vi "12 Simulated DAQmx Signal.vi"() -> ()   [LabVIEW 2017]
uses:
  <vilib>/DAQmx/configure/timing.llb/DAQmx Timing (Sample Clock).vi
  <vilib>/DAQmx/configure/trigger.llb/DAQmx Trigger.vi
  <vilib>/DAQmx/configure/trigger.llb/DAQmx Start Trigger (Digital Edge).vi
panel:
  out "Waveform Chart":dynamicdata(graph)
  in  "stop (F)":bool
  out "error out":errorcluster
  out "task out":refnum<k21>
  in  "number of samples":i32=240
  in  "rate":dbl=6000.0
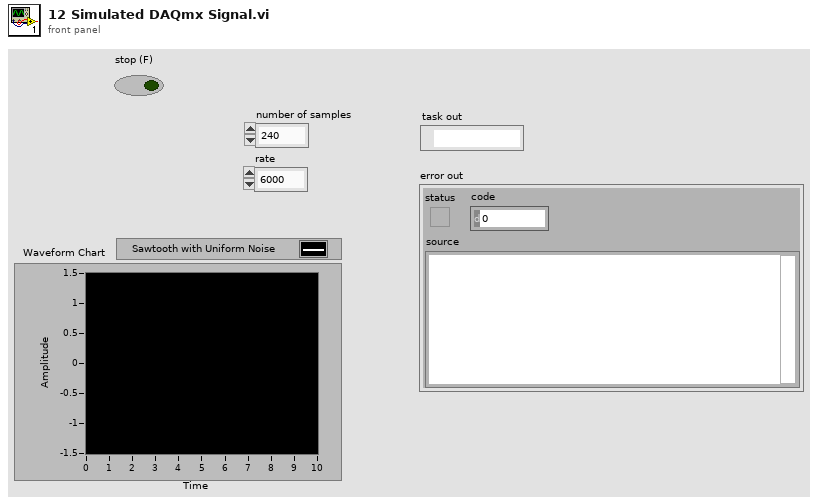
[diagram p1: front panel]
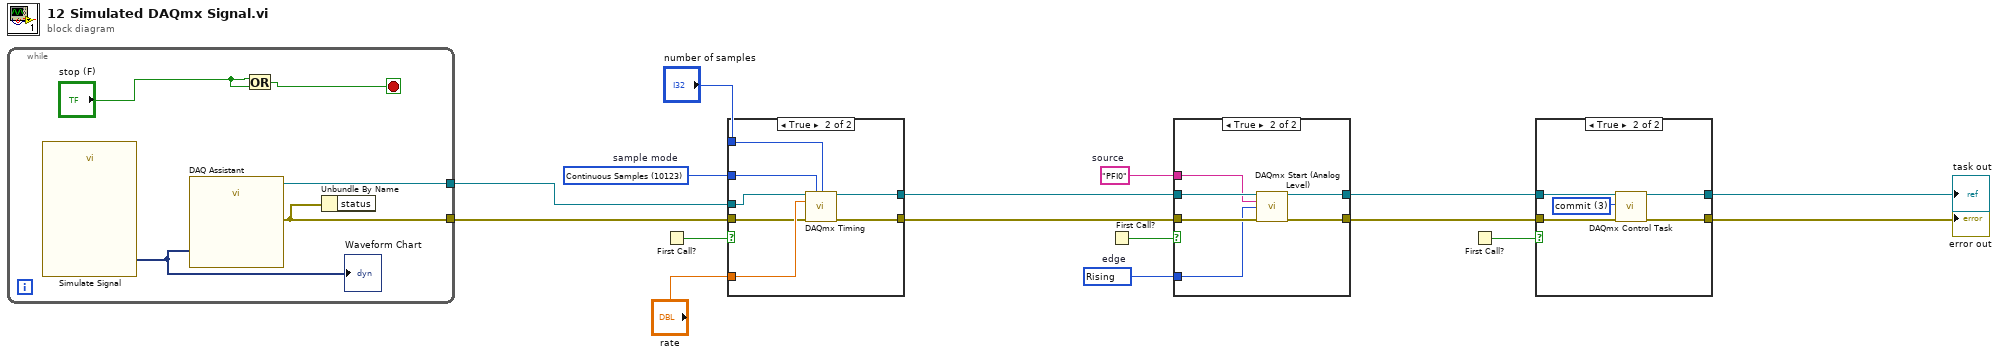
[diagram p0: block diagram]
diagram:
  w12 = 10280 items=["Rising"=10280, "Falling"=10171]  # edge
  w11 = "PFI0"  # source
  w7 = 10123 items=["Finite Samples"=10178, "Continuous Samples"=10123, "Hardware Timed Single Point"=12522]  # sample mode
  n1 = while {
    tunnel: [w20] -> w2
    tunnel: [w19] -> w1
    stop <- w21 stop-if-true
    n2 = call "Simulate Signal"() -> ("Sawtooth with Uniform Noise"=w18:dynamicdata)  [unwired: 14 in, 1 out]
    "Waveform Chart" <- w18
    n3 = call "DAQ Assistant"("data"=w18) -> ("task out"=w20:refnum<k21>, "error out"=w19:errorcluster)  [unwired: 16 in, 1 out]
    n4 = Or(x="stop (F)", y="stop (F)") -> (x .or. y?=w21:bool)
    n5 = Unbundle By Name(w19) -> ()  [unwired: 1 out]
  }
  n6 = First Call?() -> (First Call?: T/F=w3:bool)
  n7 = case shown="True" w3 {
    tunnel: [w23 w27] -> w9
    tunnel: [w22 w26] -> w4
    tunnel: "number of samples" -> [_ w30]
    tunnel: w7 -> [_ w29]
    tunnel: "rate" -> [_ w28]
    tunnel: w2 -> [w23 w25]
    tunnel: w1 -> [w22 w24]
    frame False {
    }
    frame True {
      n8 = call-poly <vilib>:"DAQmx Timing.vi"("task/channels in"=w25, "sample mode"=w29, "samples per channel"=w30, "rate"=w28, "error in"=w24) -> ("task out"=w27:refnum<k21>, "error out"=w26:errorcluster)  [unwired: 9 in]
    }
  }
  n9 = First Call?() -> (First Call?: T/F=w8:bool)
  n10 = case shown="True" w8 {
    tunnel: [w32 w36] -> w14
    tunnel: w9 -> [w32 w38]
    tunnel: [w31 w35] -> w10
    tunnel: w4 -> [w31 w37]
    tunnel: w11 -> [_ w34]
    tunnel: w12 -> [_ w33]
    frame False {
    }
    frame True {
      n11 = call-poly "DAQmx Start (Analog Level).vi"("task/channels in"=w38, "source"=w34, "edge"=w33, "error in"=w37) -> ("task out"=w36:refnum<k21>, "error out"=w35:errorcluster)  [unwired: 10 in]
    }
  }
  n12 = First Call?() -> (First Call?: T/F=w13:bool)
  n13 = case shown="True" w13 {
    tunnel: [w40 w44] -> w16
    tunnel: w14 -> [w40 w45]
    tunnel: [w39 w42] -> w15
    tunnel: w10 -> [w39 w43]
    frame False {
    }
    frame True {
      w41 = 3 items=["verify"=2, "reserve"=4, "commit"=3, "unreserve"=5, "abort"=6] ("action")
      n14 = call <vilib>:"DAQmx Control Task.vi"("task/channels in"=w45, "action"=w41, "error in"=w43) -> ("task out"=w44:refnum<k21>, "error out"=w42:errorcluster)  [unwired: 11 in]
    }
  }
  "task out" <- w16
  "error out" <- w15
